vi "Traffic Light.vi"() -> ()   [LabVIEW 2019]
panel:
  out "Hijau Bawah":bool
  out "Kuning Bawah":bool
  out "Merah Bawah":bool
  out "Hijau Kiri":bool
  out "Kuning Kiri":bool
  out "Merah Kiri":bool
  out "Hijau  Kanan":bool
  out "Kuning Kanan":bool
  out "Merah Kanan":bool
  out "Hijau Atas":bool
  out "Kuning Atas":bool
  out "Merah Atas":bool
  out "Hijau Kiri 2":bool
  out "Kuning Kiri 2":bool
  out "Merah Kiri 2":bool
  out "Hijau Bawah 2":bool
  out "Kuning Bawah 2":bool
  out "Merah Bawah 2":bool
  out "Hijau Kanan":bool
  out "Kuning Kanan 2":bool
  out "Merah Kanan 2":bool
  out "Hijau Atas 2":bool
  out "Kuning Atas 2":bool
  out "Merah Atas 2":bool
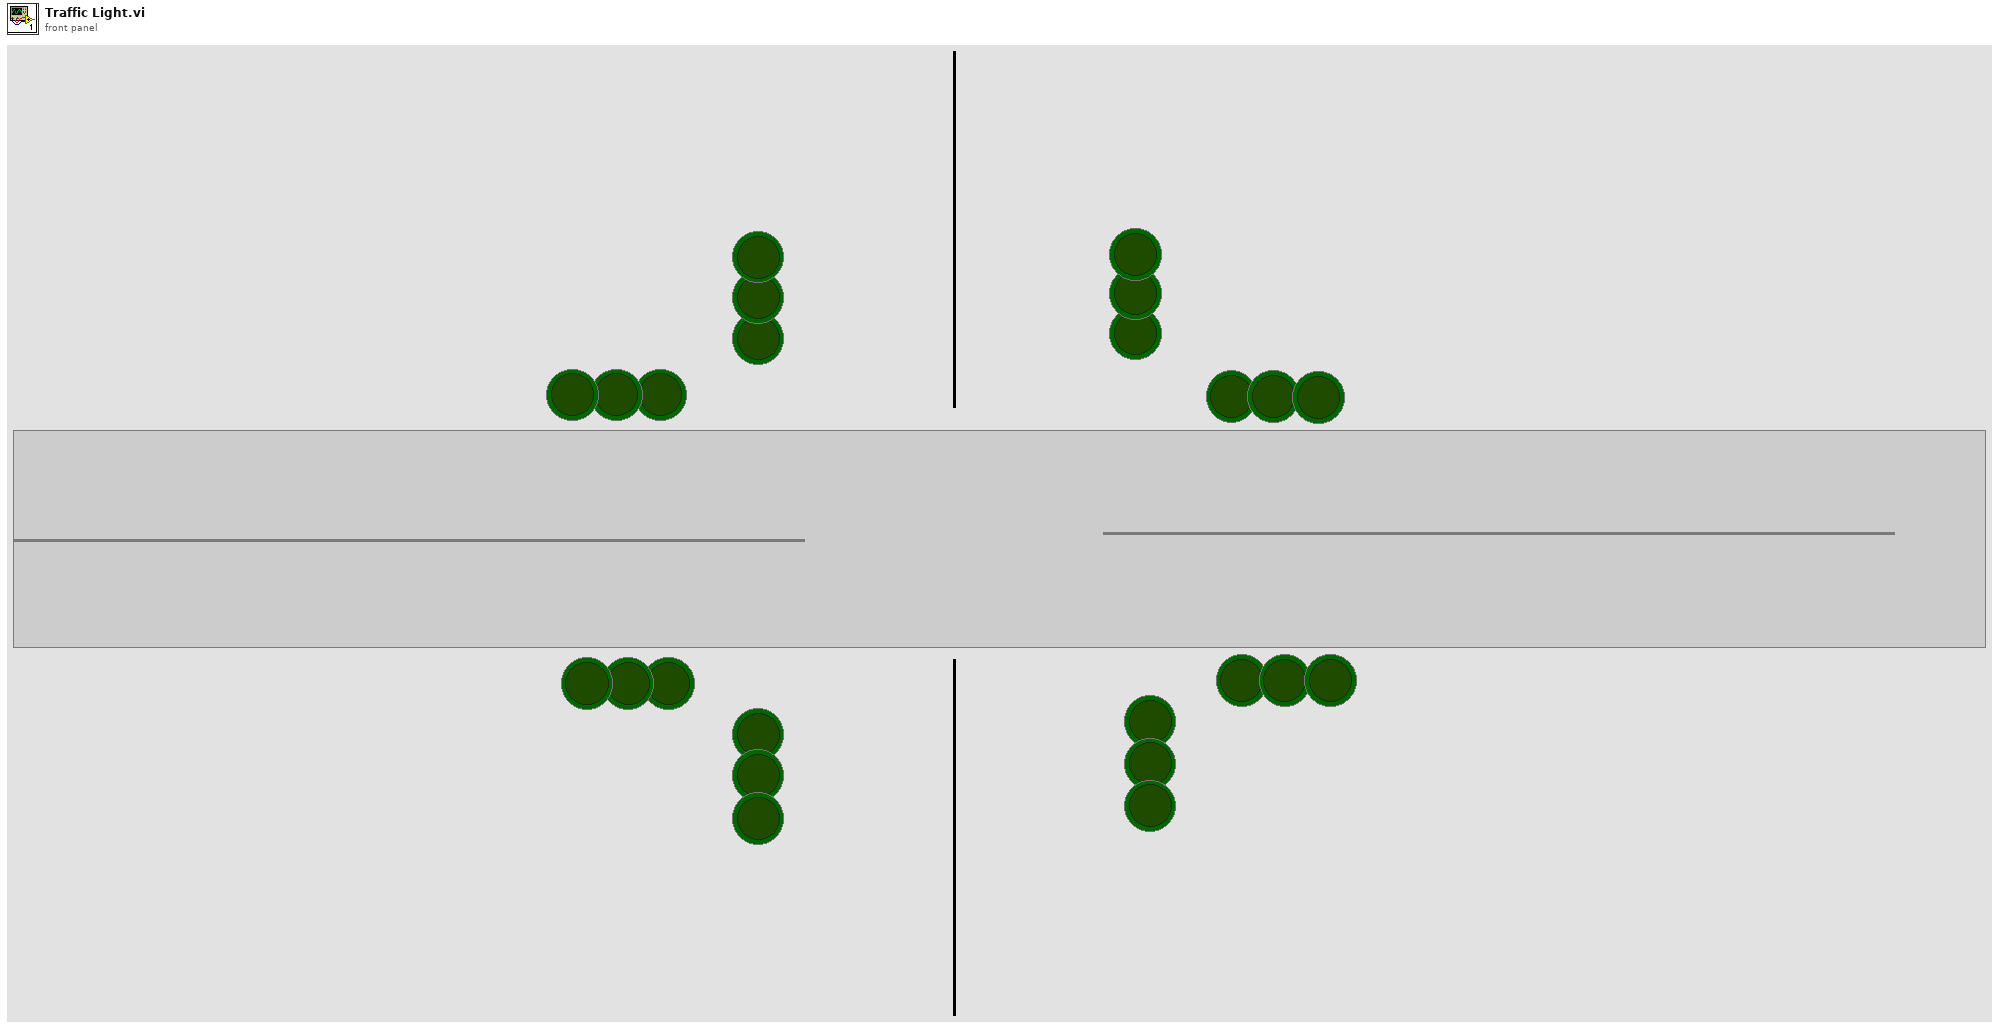
[diagram p1: front panel]
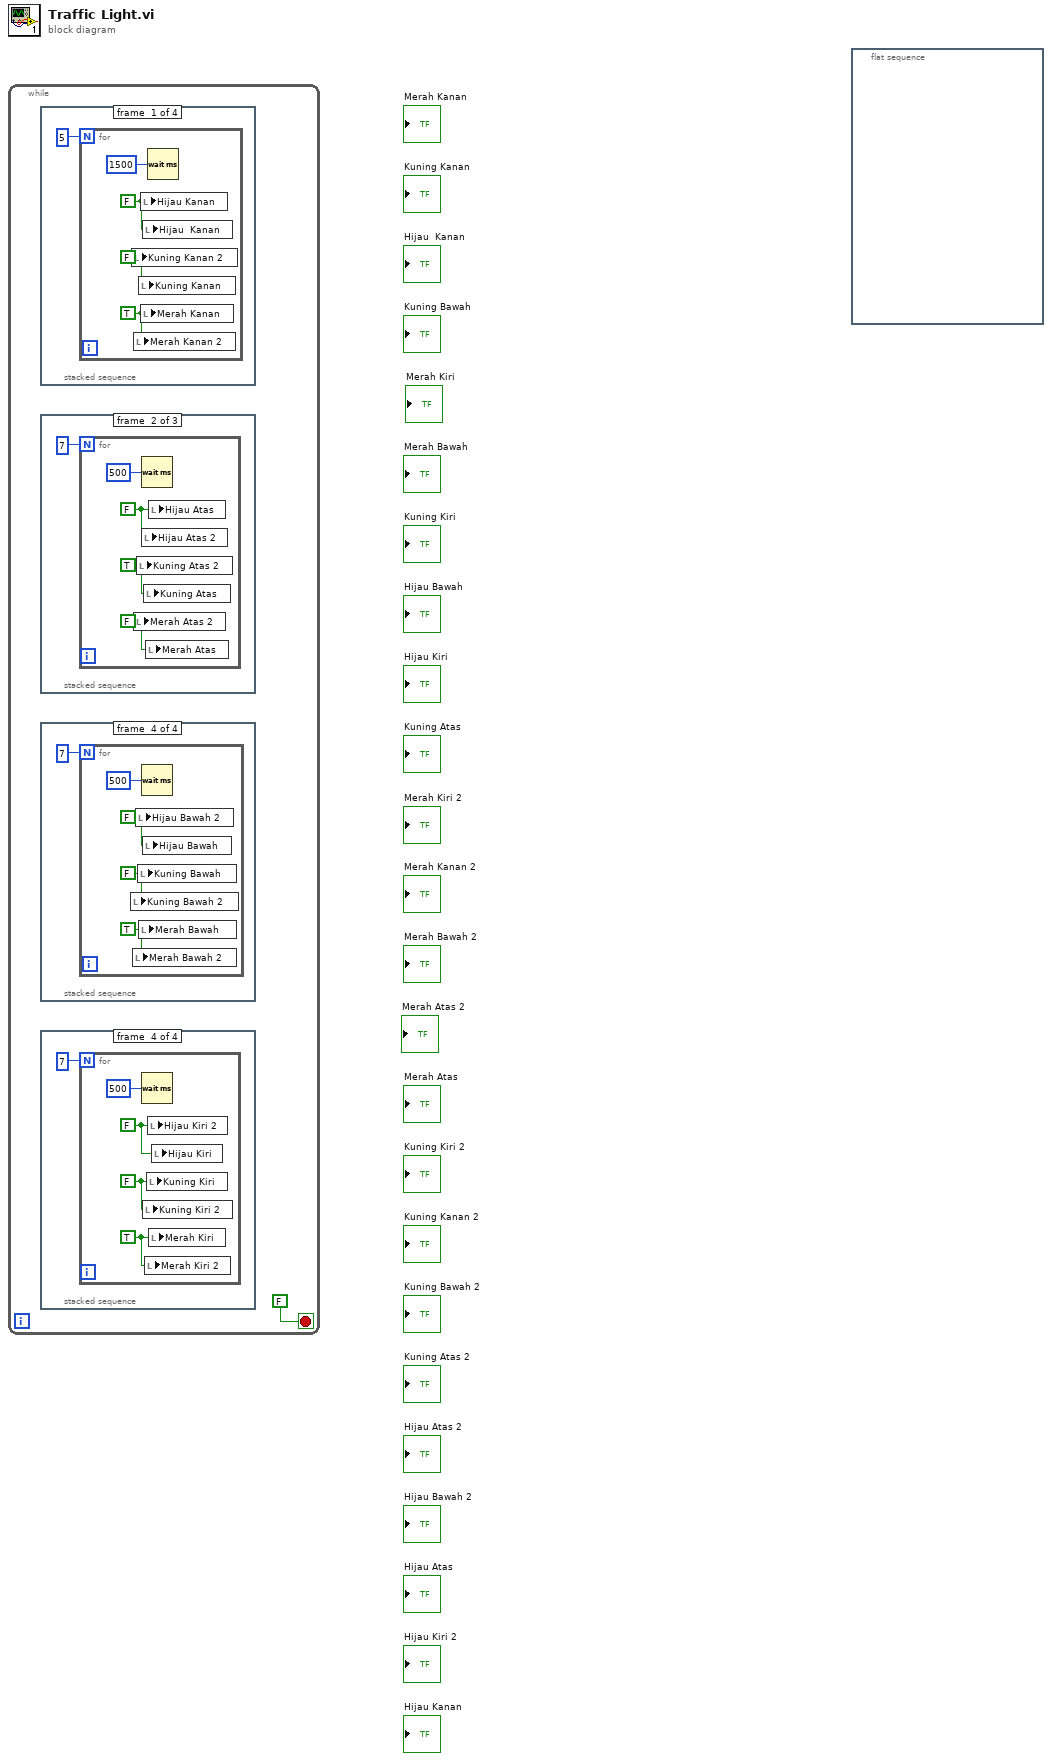
[diagram p0: block diagram]
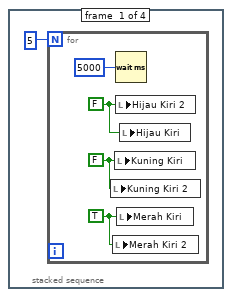
[diagram p2: hidden frame]
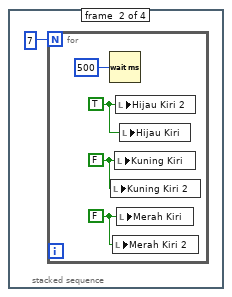
[diagram p3: hidden frame]
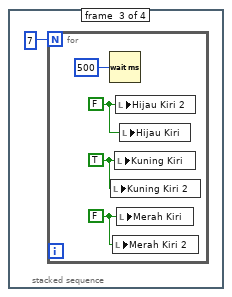
[diagram p4: hidden frame]
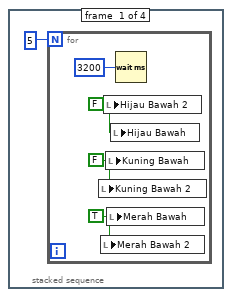
[diagram p5: hidden frame]
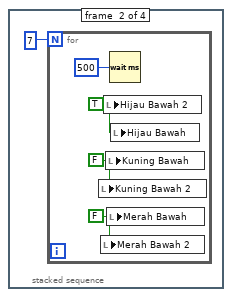
[diagram p6: hidden frame]
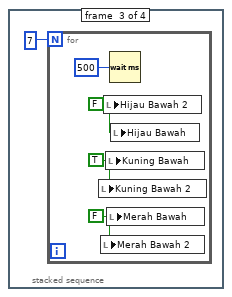
[diagram p7: hidden frame]
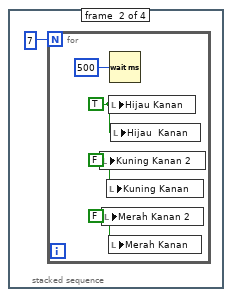
[diagram p8: hidden frame]
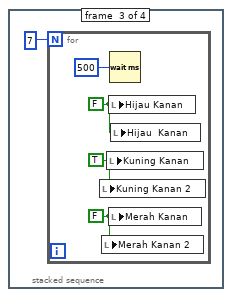
[diagram p9: hidden frame]
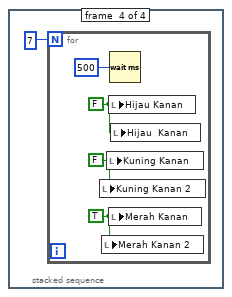
[diagram p10: hidden frame]
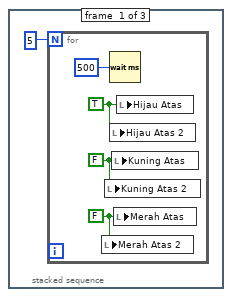
[diagram p11: hidden frame]
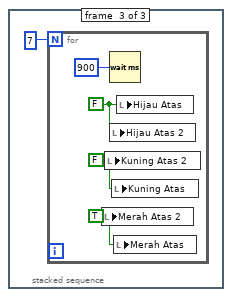
[diagram p12: hidden frame]
diagram:
  n1 = while {
    stop <- FALSE stop-if-true
    n2 = stacked-sequence {
      frame #0 {
        n3 = for {
          N: 5 -> [_]
          w43 = FALSE ("Boolean 3")
          w44 = FALSE ("Boolean 2")
          w45 = TRUE ("Boolean")
          n4 = local write "Kuning Kanan 2"(w44) -> ()
          n5 = local write "Merah Kanan 2"(w45) -> ()
          n6 = local write "Kuning Kanan"(w44) -> ()
          n7 = local write "Hijau Kanan"(w43) -> ()
          n8 = local write "Merah Kanan"(w45) -> ()
          n9 = local write "Hijau  Kanan"(w43) -> ()
          n10 = Wait (ms)(milliseconds to wait=u32 1500) -> ()  [unwired: 1 out]
        }
      }
      frame #1 {
        n11 = for {
          N: 7 -> [_]
          w48 = TRUE ("Boolean 3")
          w49 = FALSE ("Boolean 2")
          w50 = FALSE ("Boolean")
          n12 = local write "Kuning Kanan 2"(w49) -> ()
          n13 = local write "Merah Kanan 2"(w50) -> ()
          n14 = local write "Kuning Kanan"(w49) -> ()
          n15 = local write "Hijau Kanan"(w48) -> ()
          n16 = local write "Merah Kanan"(w50) -> ()
          n17 = Wait (ms)(milliseconds to wait=u32 500) -> ()  [unwired: 1 out]
          n18 = local write "Hijau  Kanan"(w48) -> ()
        }
      }
      frame #2 {
        n19 = for {
          N: 7 -> [_]
          w53 = FALSE ("Boolean 3")
          w54 = TRUE ("Boolean 2")
          w55 = FALSE ("Boolean")
          n20 = local write "Kuning Kanan 2"(w54) -> ()
          n21 = local write "Merah Kanan 2"(w55) -> ()
          n22 = local write "Kuning Kanan"(w54) -> ()
          n23 = local write "Hijau Kanan"(w53) -> ()
          n24 = local write "Merah Kanan"(w55) -> ()
          n25 = Wait (ms)(milliseconds to wait=u32 500) -> ()  [unwired: 1 out]
          n26 = local write "Hijau  Kanan"(w53) -> ()
        }
      }
      frame #3 {
        n27 = for {
          N: 7 -> [_]
          w58 = FALSE ("Boolean 3")
          w59 = FALSE ("Boolean 2")
          w60 = TRUE ("Boolean")
          n28 = local write "Kuning Kanan 2"(w59) -> ()
          n29 = local write "Merah Kanan 2"(w60) -> ()
          n30 = local write "Kuning Kanan"(w59) -> ()
          n31 = local write "Hijau Kanan"(w58) -> ()
          n32 = local write "Merah Kanan"(w60) -> ()
          n33 = Wait (ms)(milliseconds to wait=u32 500) -> ()  [unwired: 1 out]
          n34 = local write "Hijau  Kanan"(w58) -> ()
        }
      }
    }
    n35 = stacked-sequence {
      frame #0 {
        n36 = for {
          N: 5 -> [_]
          w63 = TRUE ("Boolean 3")
          w64 = FALSE ("Boolean 2")
          w65 = FALSE ("Boolean")
          n37 = local write "Merah Atas 2"(w65) -> ()
          n38 = local write "Kuning Atas 2"(w64) -> ()
          n39 = Wait (ms)(milliseconds to wait=u32 500) -> ()  [unwired: 1 out]
          n40 = local write "Hijau Atas 2"(w63) -> ()
          n41 = local write "Kuning Atas"(w64) -> ()
          n42 = local write "Merah Atas"(w65) -> ()
          n43 = local write "Hijau Atas"(w63) -> ()
        }
      }
      frame #1 {
        n44 = for {
          N: 7 -> [_]
          w68 = FALSE ("Boolean 3")
          w69 = TRUE ("Boolean 2")
          w70 = FALSE ("Boolean")
          n45 = local write "Merah Atas 2"(w70) -> ()
          n46 = local write "Kuning Atas 2"(w69) -> ()
          n47 = Wait (ms)(milliseconds to wait=u32 500) -> ()  [unwired: 1 out]
          n48 = local write "Hijau Atas 2"(w68) -> ()
          n49 = local write "Kuning Atas"(w69) -> ()
          n50 = local write "Merah Atas"(w70) -> ()
          n51 = local write "Hijau Atas"(w68) -> ()
        }
      }
      frame #2 {
        n52 = for {
          N: 7 -> [_]
          w73 = FALSE ("Boolean 3")
          w74 = FALSE ("Boolean 2")
          w75 = TRUE ("Boolean")
          n53 = local write "Merah Atas 2"(w75) -> ()
          n54 = local write "Kuning Atas 2"(w74) -> ()
          n55 = Wait (ms)(milliseconds to wait=u32 900) -> ()  [unwired: 1 out]
          n56 = local write "Hijau Atas 2"(w73) -> ()
          n57 = local write "Kuning Atas"(w74) -> ()
          n58 = local write "Merah Atas"(w75) -> ()
          n59 = local write "Hijau Atas"(w73) -> ()
        }
      }
    }
    n60 = stacked-sequence {
      frame #0 {
        n61 = for {
          N: 5 -> [_]
          w23 = FALSE ("Boolean 3")
          w24 = FALSE ("Boolean 2")
          w25 = TRUE ("Boolean")
          n62 = local write "Kuning Bawah 2"(w24) -> ()
          n63 = local write "Merah Bawah 2"(w25) -> ()
          n64 = local write "Hijau Bawah 2"(w23) -> ()
          n65 = local write "Kuning Bawah"(w24) -> ()
          n66 = local write "Merah Bawah"(w25) -> ()
          n67 = local write "Hijau Bawah"(w23) -> ()
          n68 = Wait (ms)(milliseconds to wait=u32 3200) -> ()  [unwired: 1 out]
        }
      }
      frame #1 {
        n69 = for {
          N: 7 -> [_]
          w28 = TRUE ("Boolean 3")
          w29 = FALSE ("Boolean 2")
          w30 = FALSE ("Boolean")
          n70 = local write "Kuning Bawah 2"(w29) -> ()
          n71 = local write "Merah Bawah 2"(w30) -> ()
          n72 = local write "Hijau Bawah 2"(w28) -> ()
          n73 = local write "Kuning Bawah"(w29) -> ()
          n74 = local write "Merah Bawah"(w30) -> ()
          n75 = Wait (ms)(milliseconds to wait=u32 500) -> ()  [unwired: 1 out]
          n76 = local write "Hijau Bawah"(w28) -> ()
        }
      }
      frame #2 {
        n77 = for {
          N: 7 -> [_]
          w33 = FALSE ("Boolean 3")
          w34 = TRUE ("Boolean 2")
          w35 = FALSE ("Boolean")
          n78 = local write "Kuning Bawah 2"(w34) -> ()
          n79 = local write "Merah Bawah 2"(w35) -> ()
          n80 = local write "Hijau Bawah 2"(w33) -> ()
          n81 = local write "Kuning Bawah"(w34) -> ()
          n82 = local write "Merah Bawah"(w35) -> ()
          n83 = Wait (ms)(milliseconds to wait=u32 500) -> ()  [unwired: 1 out]
          n84 = local write "Hijau Bawah"(w33) -> ()
        }
      }
      frame #3 {
        n85 = for {
          N: 7 -> [_]
          w38 = FALSE ("Boolean 3")
          w40 = FALSE ("Boolean 2")
          w39 = TRUE ("Boolean")
          n86 = local write "Kuning Bawah 2"(w40) -> ()
          n87 = local write "Merah Bawah 2"(w39) -> ()
          n88 = local write "Hijau Bawah 2"(w38) -> ()
          n89 = local write "Kuning Bawah"(w40) -> ()
          n90 = local write "Merah Bawah"(w39) -> ()
          n91 = Wait (ms)(milliseconds to wait=u32 500) -> ()  [unwired: 1 out]
          n92 = local write "Hijau Bawah"(w38) -> ()
        }
      }
    }
    n93 = stacked-sequence {
      frame #0 {
        n94 = for {
          N: 5 -> [_]
          w3 = FALSE ("Boolean 3")
          w4 = FALSE ("Boolean 2")
          w5 = TRUE ("Boolean")
          n95 = local write "Kuning Kiri 2"(w4) -> ()
          n96 = local write "Merah Kiri 2"(w5) -> ()
          n97 = local write "Kuning Kiri"(w4) -> ()
          n98 = Wait (ms)(milliseconds to wait=u32 5000) -> ()  [unwired: 1 out]
          n99 = local write "Hijau Kiri 2"(w3) -> ()
          n100 = local write "Merah Kiri"(w5) -> ()
          n101 = local write "Hijau Kiri"(w3) -> ()
        }
      }
      frame #1 {
        n102 = for {
          N: 7 -> [_]
          w8 = TRUE ("Boolean 3")
          w9 = FALSE ("Boolean 2")
          w10 = FALSE ("Boolean")
          n103 = Wait (ms)(milliseconds to wait=u32 500) -> ()  [unwired: 1 out]
          n104 = local write "Kuning Kiri 2"(w9) -> ()
          n105 = local write "Merah Kiri 2"(w10) -> ()
          n106 = local write "Kuning Kiri"(w9) -> ()
          n107 = local write "Hijau Kiri 2"(w8) -> ()
          n108 = local write "Merah Kiri"(w10) -> ()
          n109 = local write "Hijau Kiri"(w8) -> ()
        }
      }
      frame #2 {
        n110 = for {
          N: 7 -> [_]
          w13 = FALSE ("Boolean 3")
          w14 = TRUE ("Boolean 2")
          w15 = FALSE ("Boolean")
          n111 = Wait (ms)(milliseconds to wait=u32 500) -> ()  [unwired: 1 out]
          n112 = local write "Kuning Kiri 2"(w14) -> ()
          n113 = local write "Merah Kiri 2"(w15) -> ()
          n114 = local write "Kuning Kiri"(w14) -> ()
          n115 = local write "Hijau Kiri 2"(w13) -> ()
          n116 = local write "Merah Kiri"(w15) -> ()
          n117 = local write "Hijau Kiri"(w13) -> ()
        }
      }
      frame #3 {
        n118 = for {
          N: 7 -> [_]
          w18 = FALSE ("Boolean 3")
          w19 = FALSE ("Boolean 2")
          w20 = TRUE ("Boolean")
          n119 = Wait (ms)(milliseconds to wait=u32 500) -> ()  [unwired: 1 out]
          n120 = local write "Kuning Kiri 2"(w19) -> ()
          n121 = local write "Merah Kiri 2"(w20) -> ()
          n122 = local write "Kuning Kiri"(w19) -> ()
          n123 = local write "Hijau Kiri 2"(w18) -> ()
          n124 = local write "Merah Kiri"(w20) -> ()
          n125 = local write "Hijau Kiri"(w18) -> ()
        }
      }
    }
  }
  n126 = flat-sequence {
    frame #0 {
    }
  }
